vi "Users UI.vi"() -> ()   [LabVIEW 2009, in "UI.lvlib"]
uses:
  UI.lvlib
panel:
  in  "Delete":bool
  in  "Create":bool
  in  "Users List":i32(listbox)
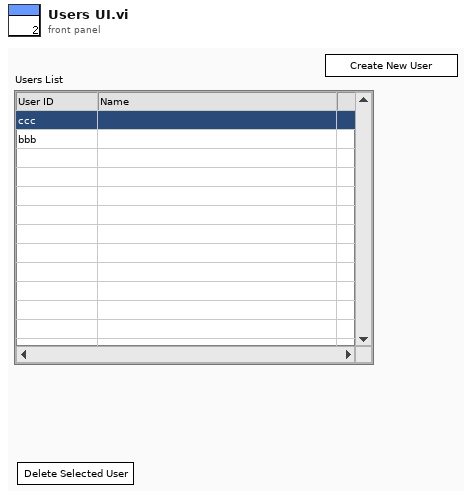
[diagram p1: front panel]
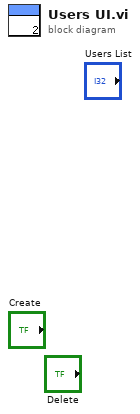
[diagram p0: block diagram]
diagram:
